vi "Rotate PID.vi"(11 "Degrees":dbl=-120.0 format="%#_13g") -> ()   [LabVIEW 2015]
uses:
  Sprocket/src/Action/Action Name.ctl
  Drive/Drive States.ctl
  Sprocket/src/Refname/Refname to String.vi
  Sprocket/src/Refname/Refname to String (Queue).vi
  Sprocket/src/Stream/Obtain Stream.vi
  Sprocket/src/Stream/Push Stream.vi
  Sprocket/src/Stream/Release Stream.vi
  Main/Robot Global Data.vi
  Sprocket/lib/Sprocket.lvlib
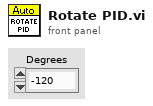
[diagram p1: front panel]
types:
  T1 = typedef "Sprocket.lvlib/Action Name.ctl" = enum16{"No Action", "Drive Train Both", "Drive Train Rotate", "Drive Train Throttle", "Collector Motor Roll", "Collector Motor Eject", "Collector Motor Collect", "Collector Motor Stop", "Collector Extend", "Collector Retract", "Shifter High", "Shifter Low", "Collector Motor Stall", "Wedge Roll"}
  T2 = typedef "Drive States.ctl" = enum16{"Idle", "Teleop", "Start Rotate", "Do Rotate", "Stop Rotate", "Start Throttle", "Do Throttle", "Stop Throttle"}
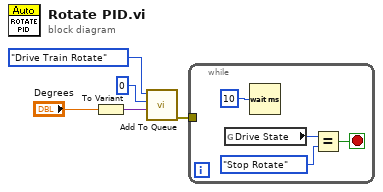
[diagram p0: block diagram]
diagram:
  n1 = To Variant(anything="Degrees") -> (Variant=w3:variant)
  n2 = call "Add To Queue.vi"("Data"=w3, "Priority"=0, "Action"=Action_Name."Drive Train Rotate") -> ("error out"=w1:errorcluster)  [unwired: 8 in]
  n3 = while {
    tunnel: w1 -> [_]
    stop <- w8 stop-if-true
    n4 = global read "Robot Global Data.vi" "Drive State"() -> (w9:T2)
    n5 = Wait (ms)(milliseconds to wait=u32 10) -> ()  [unwired: 1 out]
    n6 = Equal?(x=w9, y=Drive_States."Stop Rotate" ("t")) -> (x = y?=w8:bool)
  }
